vi "Motor Controllervi.vi"(0 "Up Limit":bool, 1 "Down Limit":bool, 2 "Left Limit":bool, 3 "Right Limit":bool, 5 "Down":bool, 7 "f":dbl, 9 "Up":bool, 12 "Left":bool, 13 "Right\n in":bool, 14 "f 2":dbl) -> (4 "Numeric 2":dbl, 6 "Numeric":dbl)   [LabVIEW 2015]
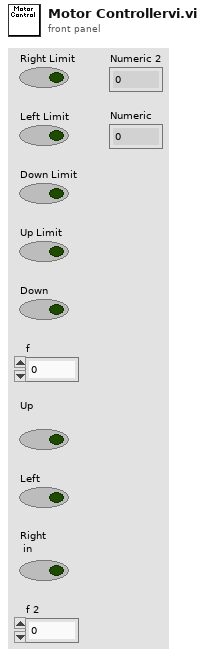
[diagram p1: front panel]
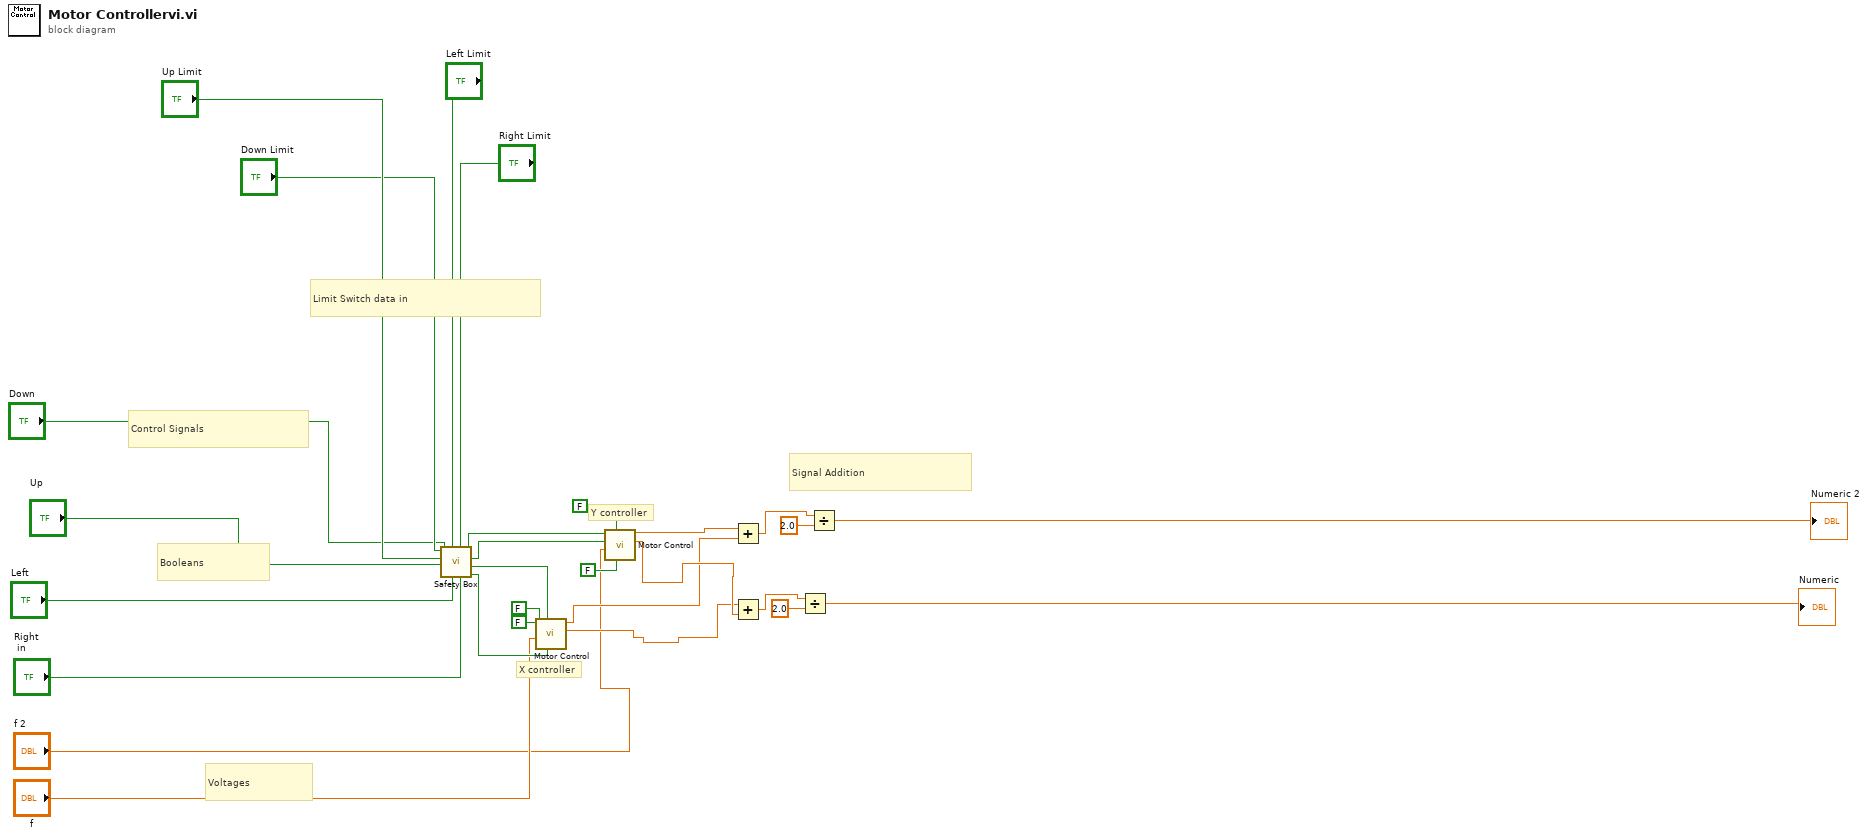
[diagram p0: block diagram]
diagram:
  # "Signal Addition"
  # "Voltages"
  # "Booleans"
  # "Control Signals"
  # "Limit Switch data in"
  # "X controller"
  # "Y controller"
  n1 = call "Safety Box.vi"("Right\n in"="Right\n in", "Left Limit In"="Right Limit", "Left in"="Left", "Right Limit"="Left Limit", "Up in"="Up", "Down in"="Down", "Up Limit"="Up Limit", "Down limit"="Down Limit") -> ("Left out"=w25:bool, "Right out"=w26:bool, "Up Out"=w24:bool, "Down out"=w23:bool)
  n2 = call "Motor Control.vi"("Left"=w25, "Right"=w26, "Voltage"="f", "Up"=FALSE, "Down"=FALSE) -> ("Motor 1"=w15:dbl, "Motor 2"=w16:dbl)  [unwired: 5 in]
  n3 = call "Motor Control.vi"("Left"=FALSE, "Right"=FALSE, "Voltage"="f 2", "Up"=w24, "Down"=w23) -> ("Motor 1"=w18:dbl, "Motor 2"=w17:dbl)  [unwired: 5 in]
  n4 = Add(x=w17, y=w16) -> (x+y=w22:dbl)
  n5 = Add(x=w15, y=w18) -> (x+y=w21:dbl)
  n6 = Divide(x=w21, y=2.0) -> (x/y=→"Numeric":dbl)
  n7 = Divide(x=w22, y=2.0) -> (x/y=→"Numeric 2":dbl)
